vi "FF Calibration Report.vi"(8 "error in (no error)":errorcluster, 9 "pass_or_fail":string, 10 "operator_name":string="Kiran", 11 "Instrument_serial Number":string="021099") -> (0 "error out":errorcluster, 3 "return value":string)   [LabVIEW 2025]
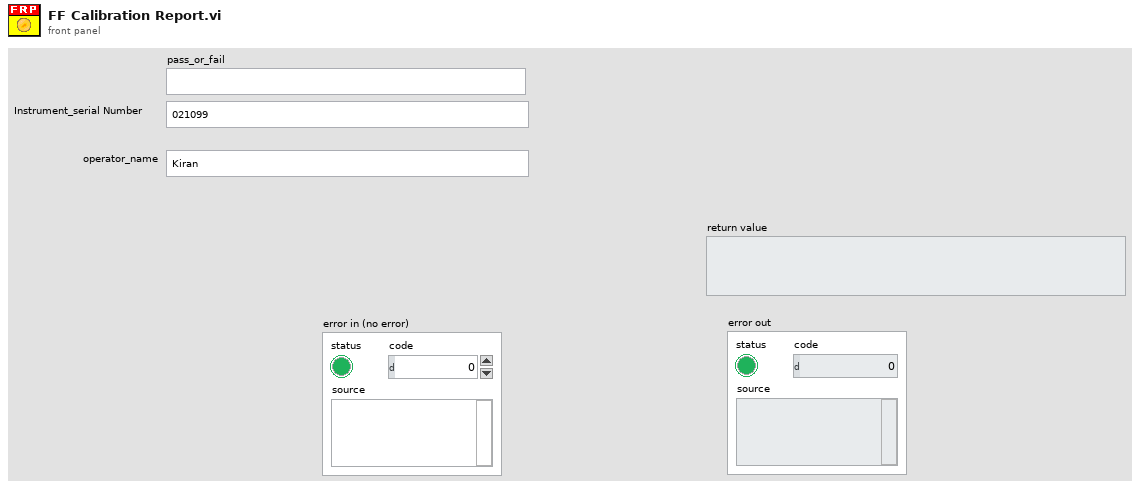
[diagram p1: front panel]
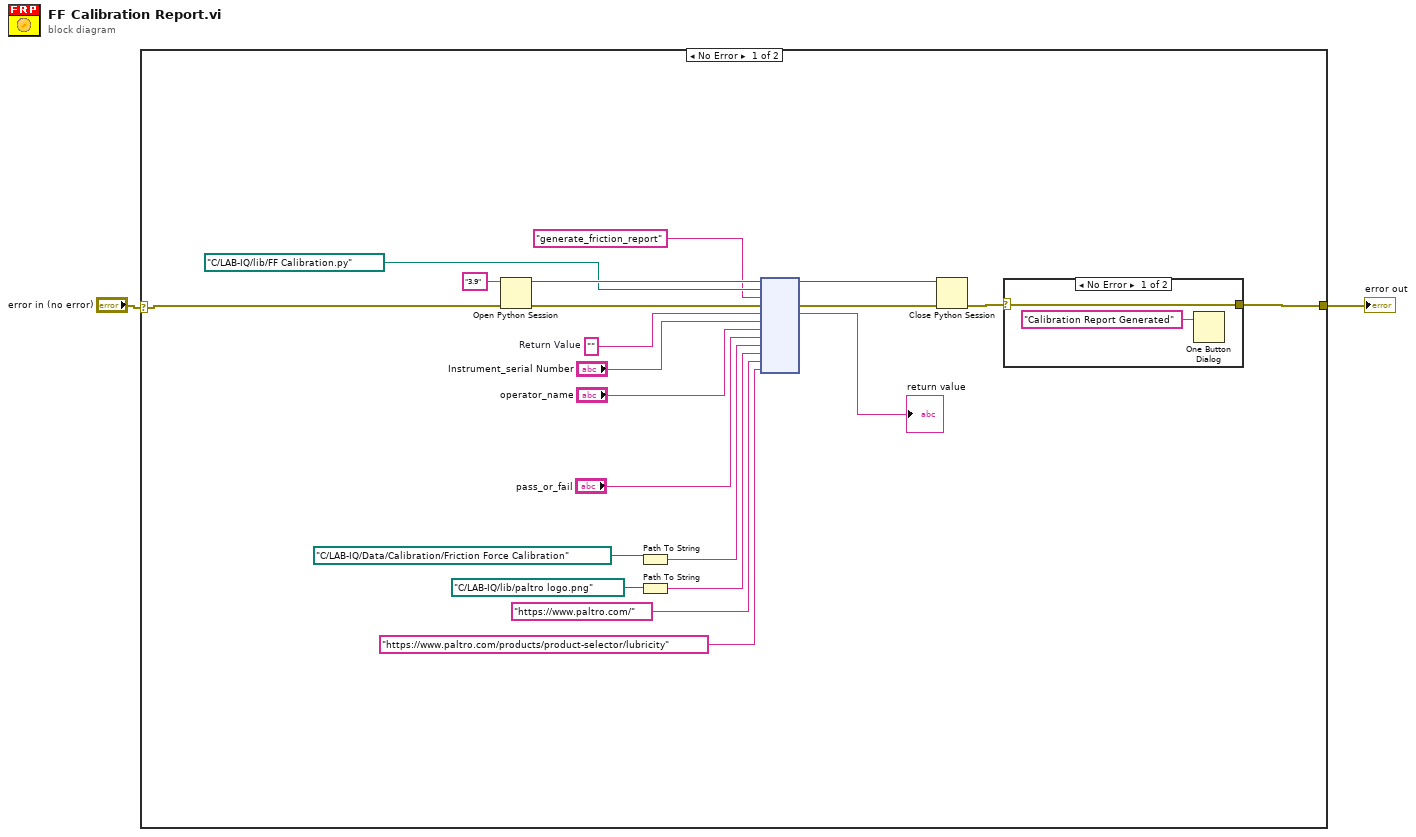
[diagram p0: block diagram]
diagram:
  n1 = case shown="No Error" "error in (no error)" {
    selector: "error in (no error)" -> [w10 _]
    tunnel: [w8 _] -> w2
    frame No Error {
      w18 = ""  # Return Value
      n2 = Open Python Session(python version="3.9" ("Python version"), 3:w10) -> (session out=w22:refnum<k35>, error out=w21:errorcluster)  [unwired: 1 in]
      n3 = Path To String(path=path "C:/LAB-IQ/Data/Calibration/Friction Force Calibration" ("output_dir")) -> (string=w6:string)
      n4 = Path To String(path=path "C:/LAB-IQ/lib/paltro logo.png" ("logo_path")) -> (string=w5:string)
      n5 = node(w22, path "C:/LAB-IQ/lib/FF Calibration.py" ("Python path"), "generate_friction_report" ("function name"), w21, w18, "Instrument_serial Number", "operator_name", "pass_or_fail", w6, w5, "https://www.paltro.com/" ("logo_link_url"), "https://www.paltro.com/products/product-selector/lubricity" ("footer_link_url")) -> (w11:refnum<k35>, w12:errorcluster, →"return value":string)  [unwired: 7 in, 2 out]
      n6 = Close Python Session(session in=w11, error in=w12) -> (11:w9:errorcluster)
      n7 = case shown="No Error" w9 {
        selector: w9 -> [w25 _]
        tunnel: [w25 _] -> w8
        frame No Error {
          n8 = One Button Dialog(message="Calibration Report Generated") -> ()  [unwired: 1 in, 1 out]
        }
        frame Error {
        }
      }
    }
    frame Error {
    }
  }
  "error out" <- w2
